vi "humiditySensor_Init.vi"(8 "error in (no error)":errorcluster, 11 "humiditySensor in":refnum<class "humiditySensor.lvclass">) -> (0 "error out":errorcluster, 3 "humiditySensor out":refnum<class "humiditySensor.lvclass">)   [LabVIEW 2020, in "RPI.SenseHat.Sensors.lvlib" / "humiditySensor.lvclass"]
uses:
  humiditySensor.lvclass
  humiditySensor.lvclass/humiditySensor.ctl
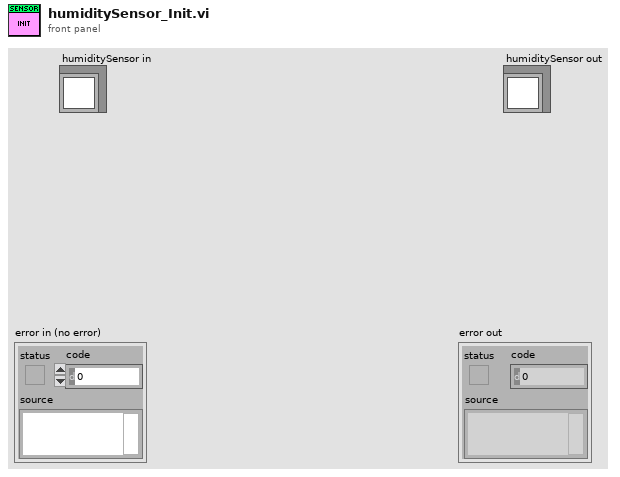
[diagram p1: front panel]
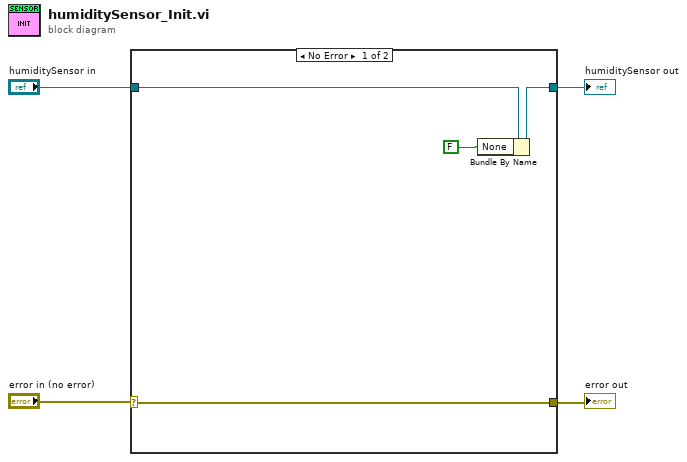
[diagram p0: block diagram]
diagram:
  n1 = case shown="No Error" "error in (no error)" {
    selector: "error in (no error)" -> [w5 w9]
    tunnel: "humiditySensor in" -> [w8 w10]
    tunnel: [w7 w10] -> w3
    tunnel: [w5 w9] -> w1
    frame No Error {
      n2 = Bundle By Name(cluster=w8, "None"=FALSE) -> (w7:refnum<class "humiditySensor.lvclass">)
    }
    frame Error {
    }
  }
  "humiditySensor out" <- w3
  "error out" <- w1
